vi "ServiceShutdownRoutedMessage_Create.vi"(7 "Header":T1, 8 "error in (no error)":errorcluster, 10 "SendTo":string) -> (0 "error out":errorcluster, 3 "Message":T3)   [LabVIEW 2017]
uses:
  <vilib>/addons/InsightCM/MessageBus/Base/controls/Message.ctl
  <vilib>/addons/InsightCM/MessageBus/Base/controls/MessageHeader.ctl
  <vilib>/addons/InsightCM/MessageBus/Base/controls/KeyValuePair.ctl
  <vilib>/addons/InsightCM/MessageBus/Base/controls/MessageClassType.ctl
  <vilib>/addons/InsightCM/Utilities/PropertyHelpers/PropertyHelpers.lvlib
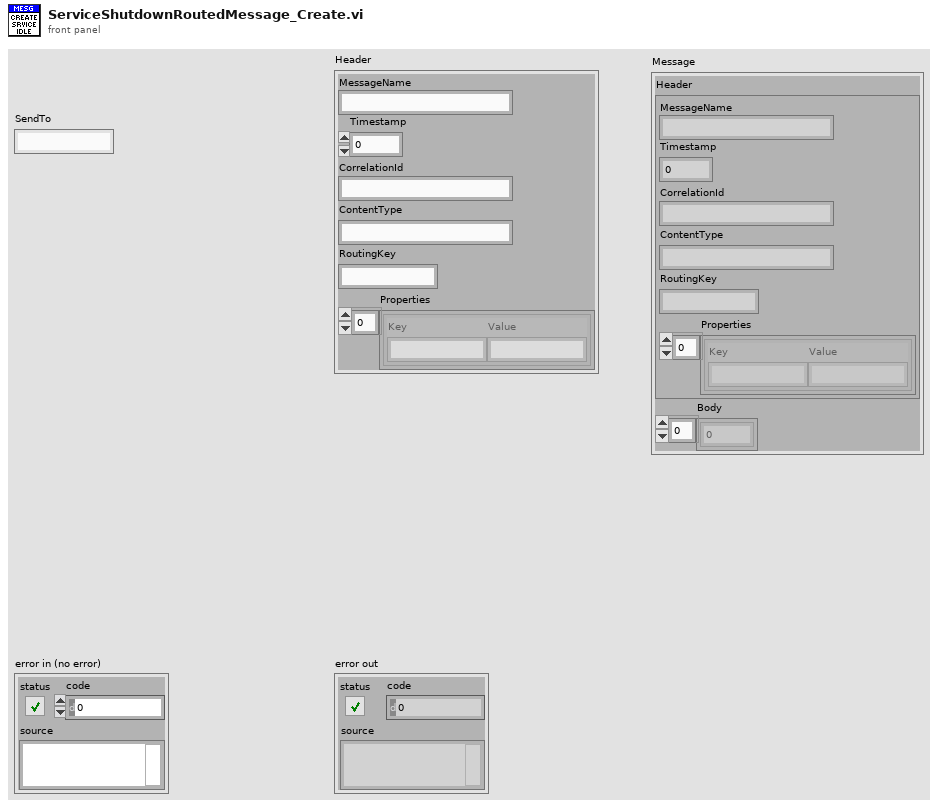
[diagram p1: front panel]
types:
  T1 = typedef "MessageHeader.ctl" = cluster{"MessageName":string, "Timestamp":i64, "CorrelationId":string, "ContentType":string, "RoutingKey":string, "Properties":T2[]}
  T2 = typedef "KeyValuePair.ctl" = cluster{"Key":string, "Value":string}
  T3 = typedef "Message.ctl" = cluster{"Header":T1, "Body":u8[]}
  T4 = typedef "MessageClassType.ctl" = enum16{"Request", "Response", "Broadcast", "RoutedMessage"}
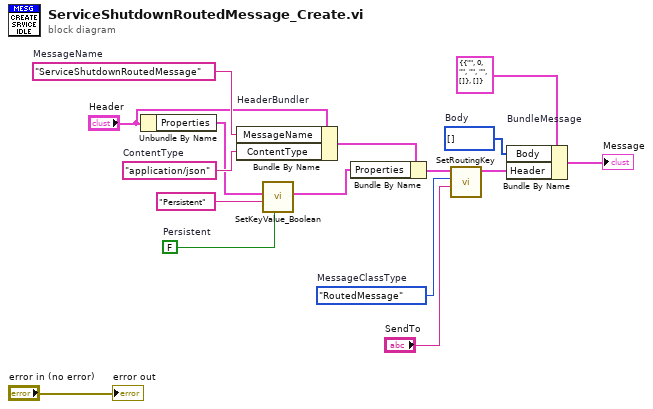
[diagram p0: block diagram]
diagram:
  w15 = u8[] []  # Body
  w13 = MessageClassType."RoutedMessage"  # MessageClassType
  w8 = FALSE  # Persistent
  w14 = "ServiceShutdownRoutedMessage"  # MessageName
  w11 = "application/json"  # ContentType
  n1 = Unbundle By Name("Header") -> ("Properties"=w10:T2[])
  n2 = Bundle By Name "HeaderBundler"(cluster="Header", "MessageName"=w14, "ContentType"=w11) -> (w5:T1)
  n3 = call <vilib>:"SetKeyValue_Boolean.vi"("value"=w8, "key"="Persistent" ("Key"), "key value pairs"=w10) -> ("key value pairs out"=w4:T2[])  [unwired: 8 in]
  n4 = Bundle By Name(cluster=w5, "Properties"=w4) -> (w6:T1)
  n5 = call <vilib>:"SetRoutingKey.vi"("SendTo"="SendTo", "MessageClassType"=w13, "Message Header in"=w6) -> ("Message Header out"=w7:T1)  [unwired: 8 in]
  n6 = Bundle By Name "BundleMessage"(cluster=T3 {"Header"={"MessageName"="", "Timestamp"=0, "CorrelationId"="", "ContentType"="", "RoutingKey"="", "Properties"=[]}, "Body"=[]} ("Message"), "Body"=w15, "Header"=w7) -> (→"Message":T3)
  "error out" <- "error in (no error)"
